vi "GetIntervalNumber.vi"(8 "error in":errorcluster, 11 "VISA resource name":refnum<visa-resource-name>) -> (0 "error out":errorcluster, 1 "Interval Number":i32, 2 "Interval Number string":string, 3 "VISA resource name out":refnum<visa-resource-name>)   [LabVIEW 2023, in "Thermotron 8800.lvlib"]
doc: "INTN\nCommand name: Send interval number\nCommand type: Program status\nDescription: Queries the 8800 for the current interval number. The 8800 sends an integer to\nindicate the interval number.\nSyntax: INTN?\nData type: Integer\nQuery example: INTN?\n8800 response: 10 (The 8800 is on interval 10 of the currently selected program.)"
uses:
  Thermotron 8800.lvlib
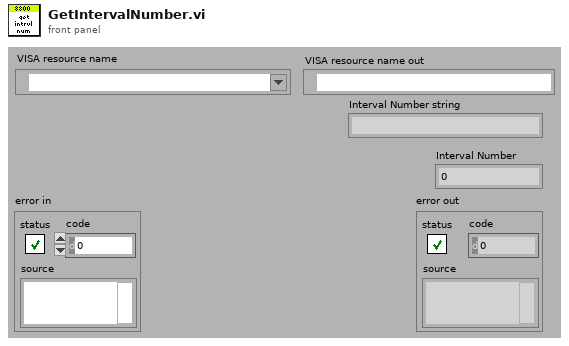
[diagram p1: front panel]
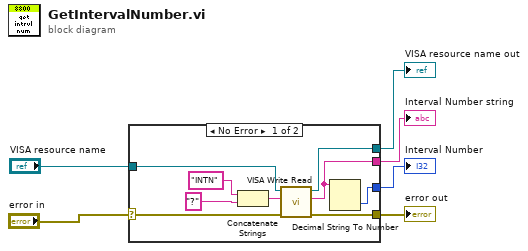
[diagram p0: block diagram]
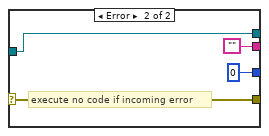
[diagram p2: hidden frame]
diagram:
  n1 = case shown="No Error" "error in" {
    selector: "error in" -> [w14 w19]
    tunnel: [w12 w19] -> w3
    tunnel: [w13 w17] -> w4
    tunnel: [w8 ""] -> w2
    tunnel: "VISA resource name" -> [w9 w17]
    tunnel: [w7 0] -> w1
    frame No Error {
      n2 = Concatenate Strings("INTN" ("8800 Command"), "?" ("8800 Command")) -> (w15:string)
      n3 = call "VISA Write Read.vi"("error in (no error)"=w14, "8800 Command"=w15, "VISA Refnum in"=w9) -> ("error out"=w12:errorcluster, "read buffer"=w8:string, "VISA Refnum out"=w13:refnum<visa-resource-name>)  [unwired: 6 in]
      n4 = Decimal String To Number(string=w8) -> (number=w7:i32)  [unwired: 2 in, 1 out]
    }
    frame Error {
      # "execute no code if incoming error"
    }
  }
  "VISA resource name out" <- w4
  "error out" <- w3
  "Interval Number string" <- w2
  "Interval Number" <- w1
